vi "lab2.vi"() -> ()   [LabVIEW 2014]
uses:
  <vilib>/express/express analysis/Spectral/Block/exnSpectralBlock spectral measurements RMS poly.vi
  <vilib>/express/express analysis/Spectral/Block/exnSpectralBlock spectral measurements RMS DDT.vi
  <vilib>/express/express analysis/Spectral/XNode/ExpressSpectralMeasurementsBlockNode.xnode
panel:
  out "Waveform Graph 4":dynamicdata(graph)
  out "Waveform Graph 3":dynamicdata(graph)
  out "Cycle Average":dbl
  out "Peak to Peak":dbl
  out "Waveform Graph 2":dynamicdata(graph)
  out "Waveform Graph":dynamicdata(graph)
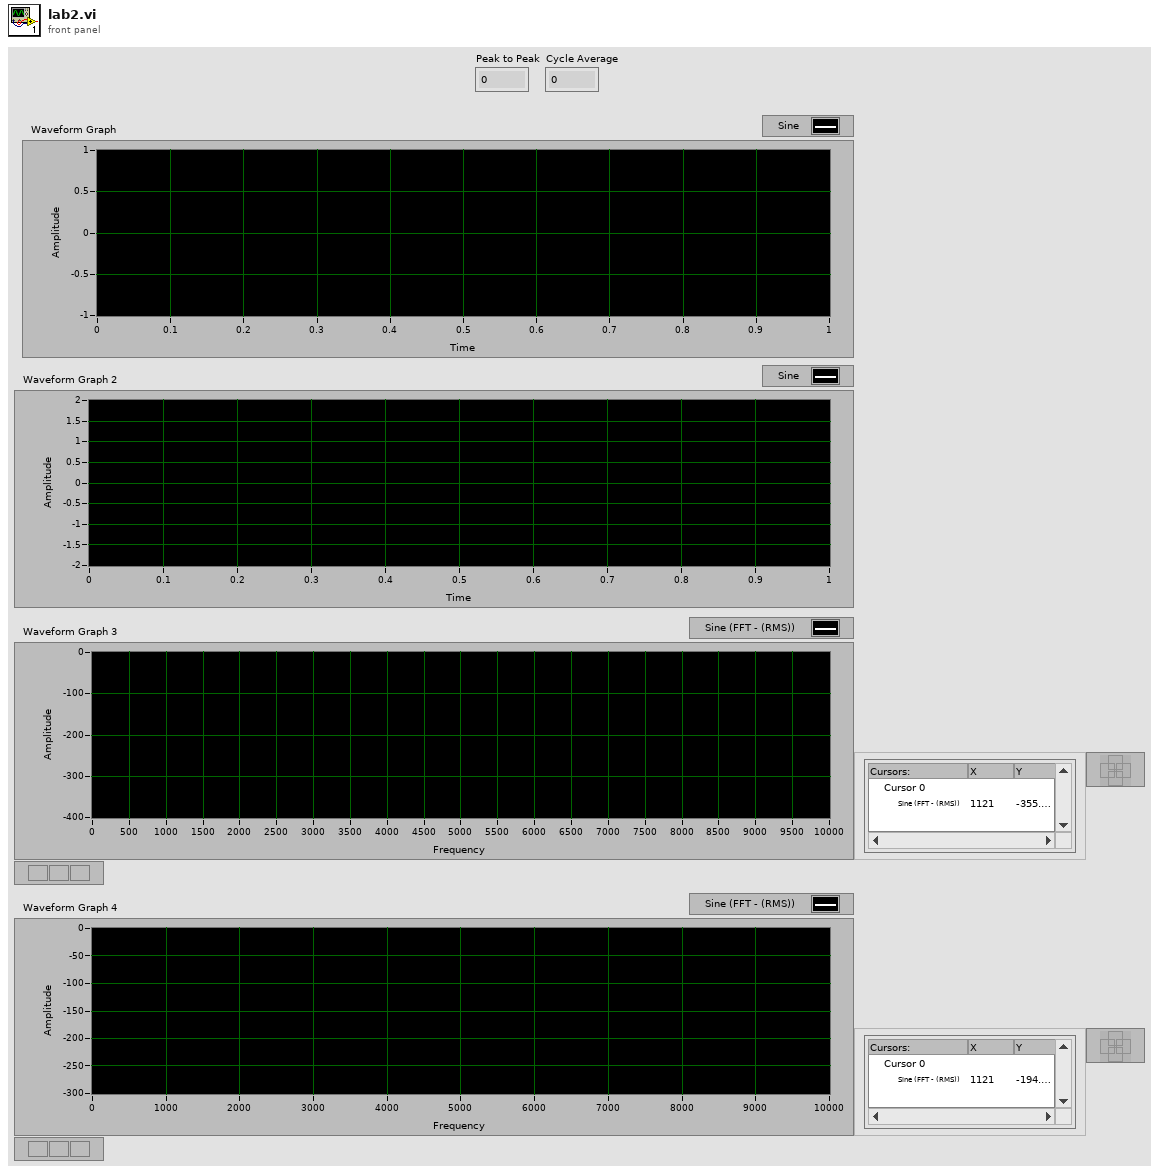
[diagram p1: front panel]
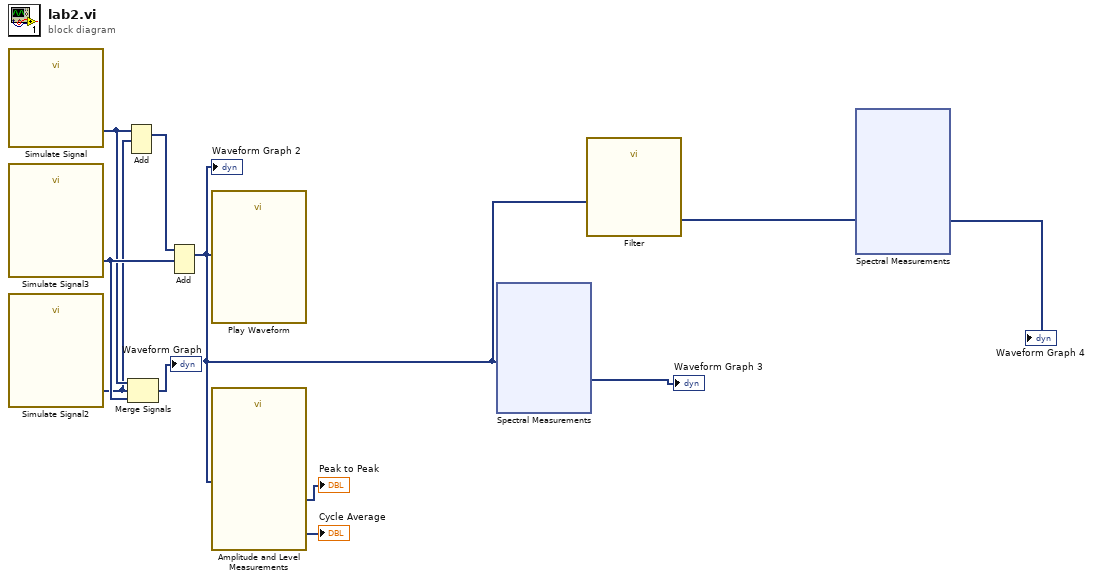
[diagram p0: block diagram]
diagram:
  n1 = call "Simulate Signal"() -> ("Sine"=w8:dynamicdata)  [unwired: 14 in, 1 out]
  n2 = call "Simulate Signal3"() -> ("Sine"=w9:dynamicdata)  [unwired: 14 in, 1 out]
  n3 = call "Simulate Signal2"() -> ("Sine"=w7:dynamicdata)  [unwired: 14 in, 1 out]
  n4 = Add(1:w7, 2:w8) -> (0:w10:dynamicdata)  [unwired: 1 in, 1 out]
  n5 = Merge Signals(w8, w7, w9) -> (→"Waveform Graph":dynamicdata)
  n6 = Add(1:w9, 2:w10) -> (0:w3:dynamicdata)  [unwired: 1 in, 1 out]
  "Waveform Graph 2" <- w3
  n7 = call "Play Waveform"("Data"=w3) -> ()  [unwired: 18 in, 1 out]
  n8 = call "Amplitude and Level Measurements"("Signals"=w3) -> ("Cycle Average"=→"Cycle Average":dynamicdata, "Peak to Peak"=→"Peak to Peak":dynamicdata)  [unwired: 12 in, 1 out]
  n9 = xnode "Spectral Measurements"("Signals"=w3) -> ("FFT - (RMS)"=→"Waveform Graph 3":dynamicdata)  [unwired: 1 in, 2 out]
  n10 = call "Filter"("Signal"=w3) -> ("Filtered Signal"=w2:dynamicdata)  [unwired: 9 in, 1 out]
  n11 = xnode "Spectral Measurements"("Signals"=w2) -> ("FFT - (RMS)"=→"Waveform Graph 4":dynamicdata)  [unwired: 1 in, 2 out]
